vi "start autotune.vi"() -> ()   [LabVIEW 2015]
panel:
  in  "period (ms)":u32=1000
  # "This VI starts all subvis for autotuning"
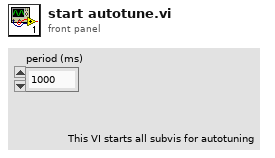
[diagram p1: front panel]
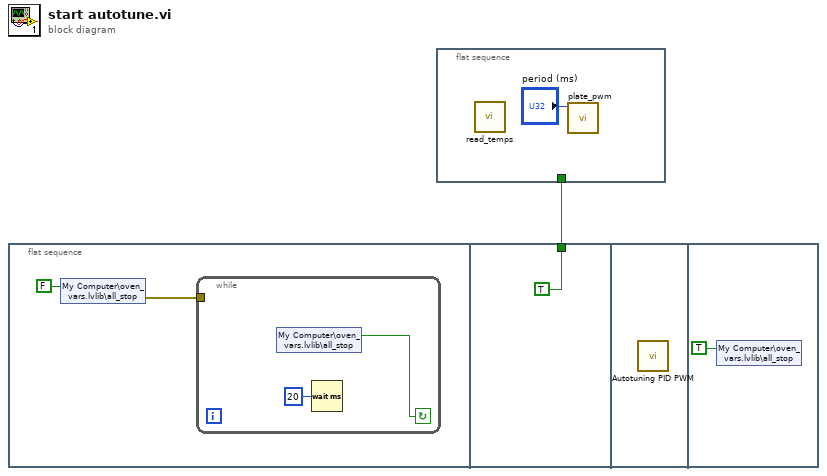
[diagram p0: block diagram]
diagram:
  n1 = flat-sequence {
    tunnel: [TRUE] -> w1
    frame #0 {
      n2 = shared-variable "My Computer\\oven_vars.lvlib\\all_stop"(FALSE ("all_stop")) -> (error out=w2:errorcluster)  [unwired: 1 in]
      n3 = while {
        tunnel: w2 -> [_]
        stop <- w5 continue-if-true
        n4 = shared-variable "My Computer\\oven_vars.lvlib\\all_stop"() -> (w5:bool)  [unwired: 1 in, 1 out]
        n5 = Wait (ms)(milliseconds to wait=u32 20) -> ()  [unwired: 1 out]
      }
    }
    frame #1 {
    }
    frame #2 {
      n6 = call "Autotuning PID PWM.vi"() -> ()  [unwired: 12 in]
    }
    frame #3 {
      n7 = shared-variable "My Computer\\oven_vars.lvlib\\all_stop"(TRUE ("all_stop")) -> ()  [unwired: 1 in, 1 out]
    }
  }
  n8 = flat-sequence {
    tunnel: w1 -> [_]
    frame #0 {
      n9 = call "read_temps.vi"() -> ()  [unwired: 12 in]
      n10 = call "plate_pwm.vi"("period (ms)"="period (ms)") -> ()  [unwired: 11 in]
    }
  }
